vi "readInTimeLabel.vi"(8 "error in (no error)":errorcluster, 10 "eventXML":refnum<k20>, 11 "Delay in":refnum<class "Delay.lvclass">) -> (0 "error out":errorcluster, 2 "eventXML out":refnum<k20>, 3 "Delay out":refnum<class "Delay.lvclass">)   [LabVIEW 2011, in "Tools.lvlib" / "Scripting.lvlib" / "Delay.lvclass"]
uses:
  Delay.lvclass
  Delay.lvclass/Delay.ctl
  <vilib>/xml/Close Reference(Node).vi
  <vilib>/xml/Close Reference(NNMap).vi
  Program Files/National Instruments/LabVIEW 2011/resource/objmgr/DOMUserDefRef.rc
  <vilib>/xml/NI_XML.lvlib
  ScriptEvent.lvclass
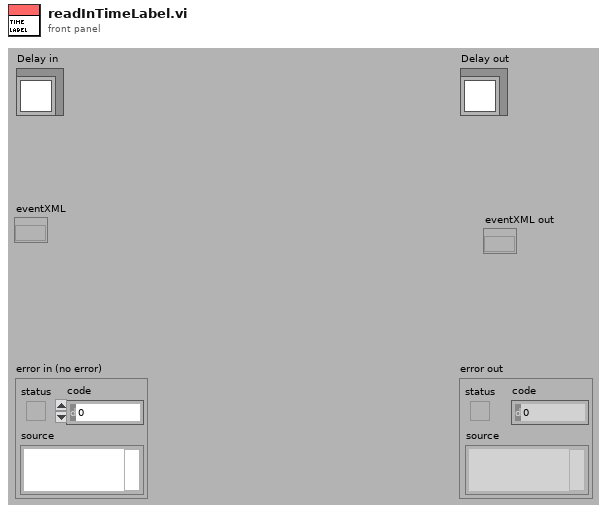
[diagram p1: front panel]
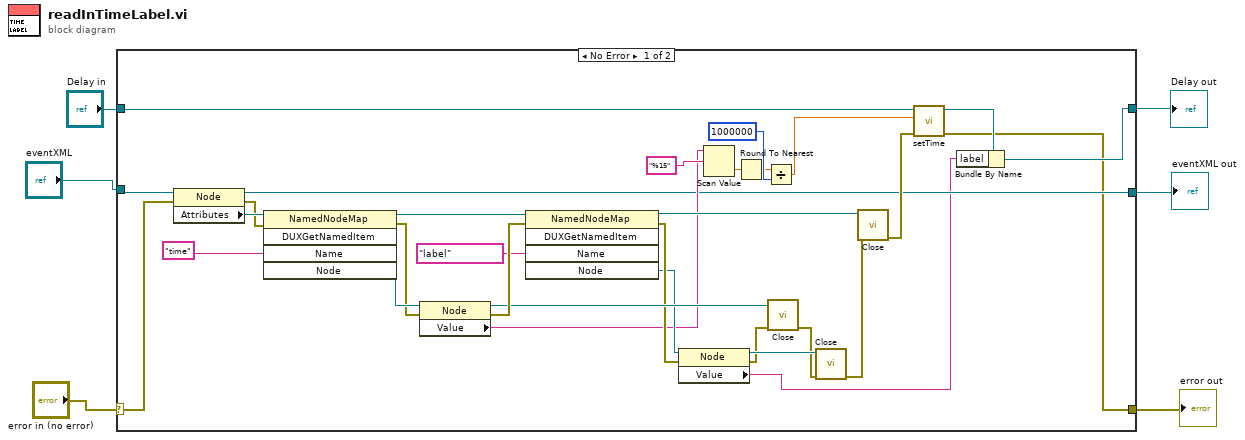
[diagram p0: block diagram]
diagram:
  n1 = case shown="No Error" "error in (no error)" {
    selector: "error in (no error)" -> [w15 w39]
    tunnel: [w9 w39] -> w1
    tunnel: [w10 w38] -> w6
    tunnel: "Delay in" -> [w16 w38]
    tunnel: "eventXML" -> [w37 _]
    tunnel: [w12 _] -> w2
    frame No Error {
      n2 = property class="Node"(reference=w37, error in=w15) -> (reference out=w12:refnum<k20>, error out=w33:errorcluster, "Attributes"=w34:refnum<k20>)
      n3 = invoke class="NamedNodeMap" method="DUXGetNamedItem"(reference=w34, error in=w33, "Name"="time") -> (reference out=w32:refnum<k20>, error out=w35:errorcluster, "Node"=w36:refnum<k20>)  [unwired: 2 in, 2 out]
      n4 = property class="Node"(reference=w36, error in=w35) -> (reference out=w30:refnum<k20>, error out=w31:errorcluster, "Value"=w19:string)
      n5 = invoke class="NamedNodeMap" method="DUXGetNamedItem"(reference=w32, error in=w31, "Name"="label") -> (reference out=w25:refnum<k20>, error out=w24:errorcluster, "Node"=w23:refnum<k20>)  [unwired: 2 in, 2 out]
      n6 = property class="Node"(reference=w23, error in=w24) -> (reference out=w29:refnum<k20>, error out=w28:errorcluster, "Value"=w8:string)
      n7 = Scan Value(string=w19, format string="%15") -> (value=w18:dbl)  [unwired: 1 in, 1 out]
      n8 = Round To Nearest(number=w18) -> (nearest integer value=w7:dbl)
      n9 = Divide(x=w7, y=1000000) -> (x/y=w14:dbl)
      n10 = call-poly <vilib>:"Close.vi"("error in (no error)"=w28, "node"=w30) -> ("error out"=w27:errorcluster)  [unwired: 7 in]
      n11 = call-poly <vilib>:"Close.vi"("error in (no error)"=w27, "node"=w29) -> ("error out"=w26:errorcluster)  [unwired: 7 in]
      n12 = call-poly <vilib>:"Close.vi"("error in (no error)"=w26, "named node map"=w25) -> ("error out"=w13:errorcluster)  [unwired: 7 in]
      n13 = call "setTime.vi"("error in (no error)"=w13, "time"=w14, "ScriptEvent.lvclass in"=w16) -> ("error out"=w9:errorcluster, "ScriptEvent.lvclass out"=w11:refnum<class "Delay.lvclass">)  [unwired: 7 in]
      n14 = Bundle By Name(cluster=w11, "label"=w8) -> (w10:refnum<class "Delay.lvclass">)
    }
    frame Error {
    }
  }
  "error out" <- w1
  "Delay out" <- w6
  "eventXML out" <- w2
